vi "Initialize New.vi"(8 "error in (no error)":errorcluster, 10 "count":i32, 11 "Core Plugins Configuration in":refnum<class "Core Plugins Configuration.lvclass">) -> (0 "error out":errorcluster, 3 "Core Plugins Configuration out":refnum<class "Core Plugins Configuration.lvclass">)   [LabVIEW 2017, in "DSF Core.lvlib" / "Core Plugins Configuration.lvclass"]
uses:
  Core Plugins Configuration.lvclass
  Typedefs/DSF Core Plugin Configuration.ctl
  Typedefs/DSF Timing Info.ctl
  Core Plugins Configuration.lvclass/Core Plugins Configuration.ctl
  DSF Core.lvlib
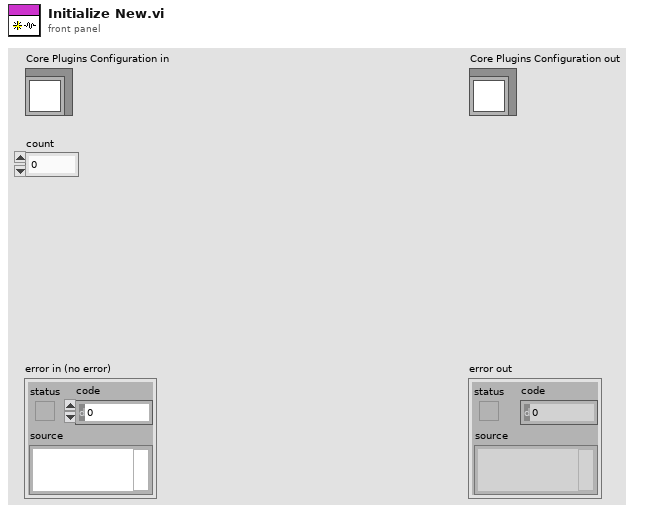
[diagram p1: front panel]
types:
  T1 = typedef "DSF Core.lvlib/DSF Core Plugin Configuration.ctl" = cluster{"name":string, "components":string[], "cycle timing":T2}
  T2 = typedef "DSF Core.lvlib/DSF Timing Info.ctl" = cluster{"priority":u64, "decimation":u64, "offset":u64}
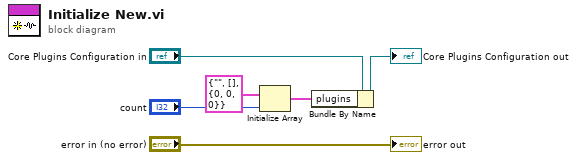
[diagram p0: block diagram]
diagram:
  n1 = Initialize Array(T1 {"name"="", "components"=[], "cycle timing"={"priority"=0, "decimation"=0, "offset"=0}} ("core plugin configuration"), "count") -> (w2:T1[])
  n2 = Bundle By Name(cluster="Core Plugins Configuration in", "plugins"=w2) -> (→"Core Plugins Configuration out":refnum<class "Core Plugins Configuration.lvclass">)
  "error out" <- "error in (no error)"
